vi "Value substituter in equations.vi"(1 "Cluster":T1={"All Param Names"=[], "All Param Values"=[], "Sp IDs"=[], "Sp States"=[], "Input Equations"=[], "CompID"=[], "CompSize"=[], "T-Sym"="time", "T"=0.0}) -> (0 "Output Equations":string[](array[string]))   [LabVIEW 2014]
doc: "This VI substitutes the numerical values of bio-model's parameters in its equations.\n\nDesigned by HB\nhaba@dtu.dk"
uses:
  ValSubsCtrl.ctl
panel:
  out "T 2":dbl
  out "CompSize 2":string[](array[string])
  out "T-Sym 2":string="time"
  out "CompID 2":string[](array[string])
  out "Input Equations 2":string[](array[string])
  out "All Param Names 2":string[](array[string])
  out "All Param Values 2":string[](array[string])
  out "Sp IDs 2":string[](array[string])
  out "Sp States 2":string[](array[string])
  out "operators (none)":string[](array[string])=["*", "+", "-", "/", "^", "(", ")"]
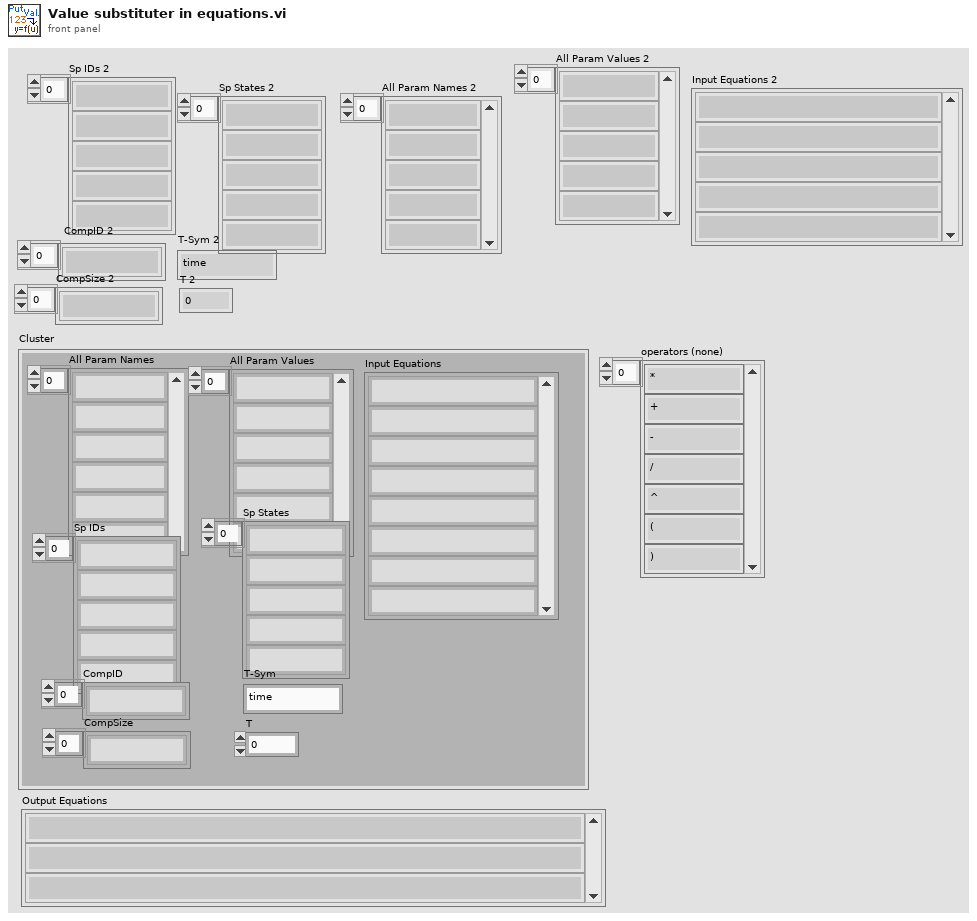
[diagram p1: front panel]
types:
  T1 = typedef "ValSubsCtrl.ctl" = cluster{"All Param Names":string[], "All Param Values":string[], "Sp IDs":string[], "Sp States":string[], "Input Equations":string[], "CompID":string[], "CompSize":string[], "T-Sym":string, "T":dbl}
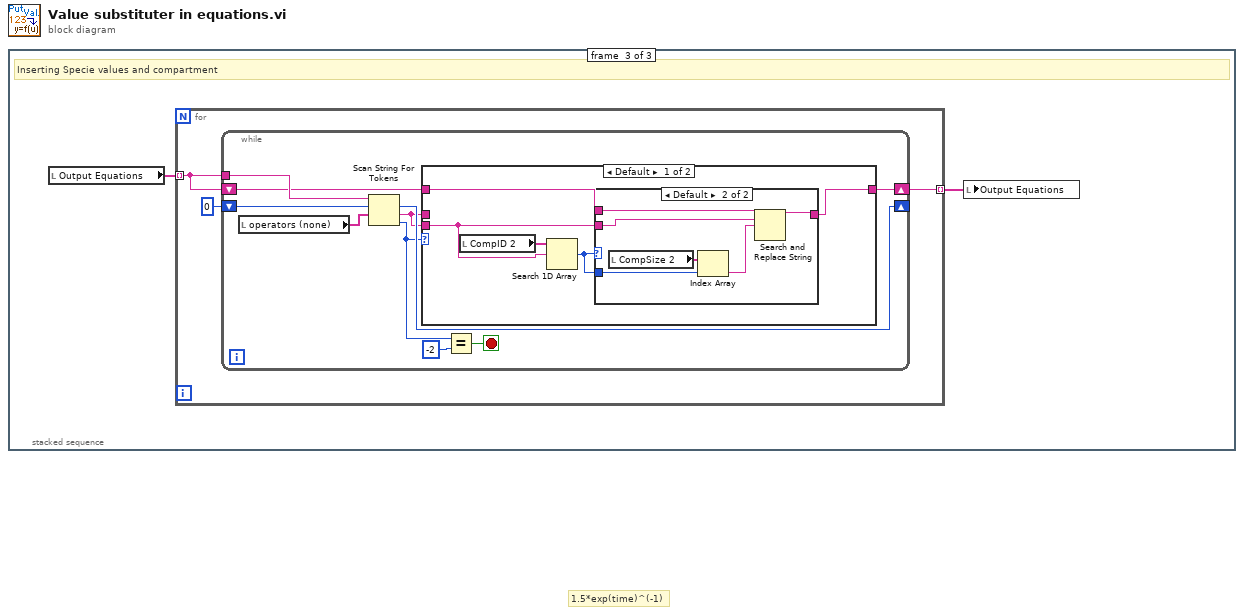
[diagram p0: block diagram]
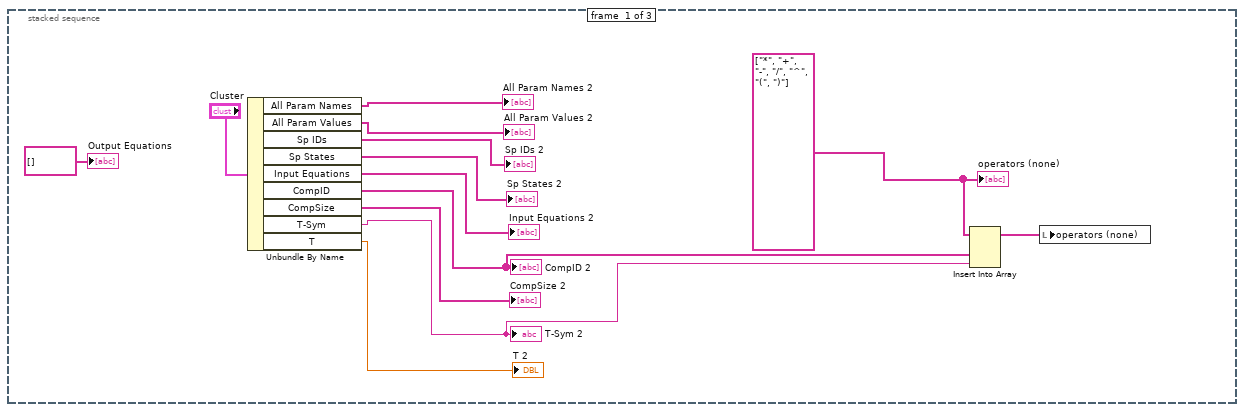
[diagram p2: hidden frame]
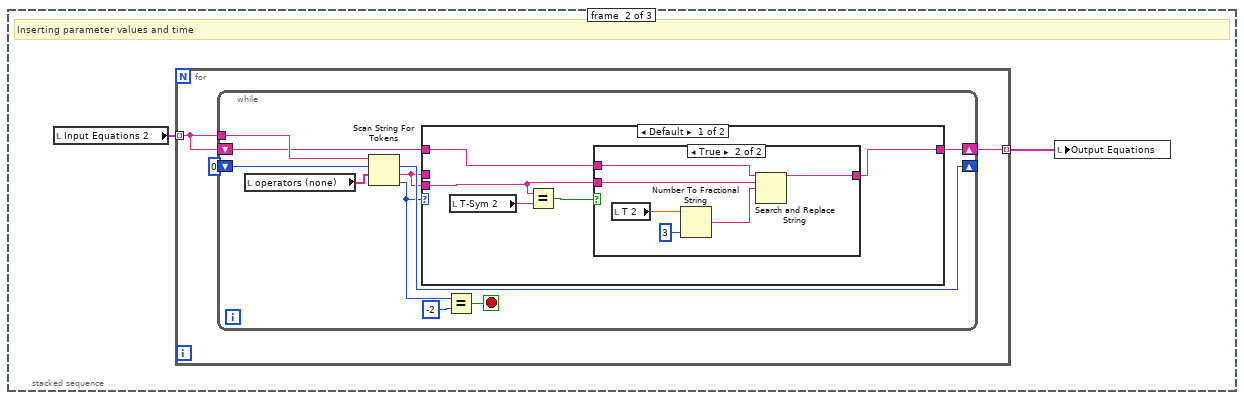
[diagram p3: hidden frame]
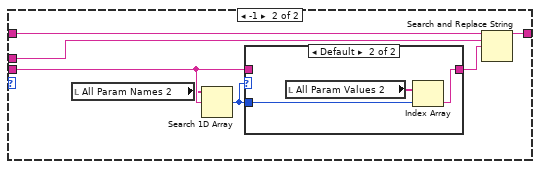
[diagram p5: hidden frame]
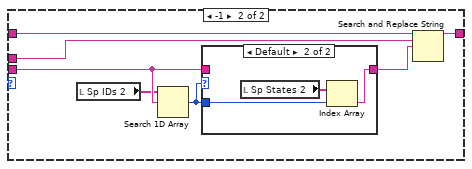
[diagram p8: hidden frame]
diagram:
  # "1.5*exp(time)^(-1)"
  n1 = stacked-sequence {
    frame #0 {
      w12 = string[] ["*", "+", "-", "/", "^", "(", ")"] ("operators (none)")
      n2 = Unbundle By Name("Cluster") -> ("All Param Names"=→"All Param Names 2":string[], "All Param Values"=→"All Param Values 2":string[], "Sp IDs"=→"Sp IDs 2":string[], "Sp States"=→"Sp States 2":string[], "Input Equations"=→"Input Equations 2":string[], "CompID"=w3:string[], "CompSize"=→"CompSize 2":string[], "T-Sym"=w2:string, "T"=→"T 2":dbl)
      "CompID 2" <- w3
      "T-Sym 2" <- w2
      n3 = Insert Into Array(array=w12, new element #1=w3, new element #2=w2) -> (w11:string[])  [unwired: 1 in]
      n4 = local write "operators (none)"(w11) -> ()
      "Output Equations" <- string[] [] ("Output Equations")
      "operators (none)" <- w12
    }
    frame #1 {
      # "Inserting parameter values and time"
      n5 = local read "Input Equations 2"() -> (w15:string[])
      n6 = for {
        tunnel: w15 -> [w17] mode=indexing
        tunnel: [w16] -> w14 mode=indexing
        n7 = while {
          shift-right: [w25] -> _
          shift-left: 0 ("offset past token") -> [w28]
          shift-right: [w20] -> w16
          shift-left: w17 -> [w21]
          tunnel: w17 -> [w22]
          stop <- w26 stop-if-true
          n8 = local read "operators (none)"() -> (w19:string[])
          n9 = Scan String For Tokens(7:w19, 8:w28, 9:w22) -> (0:w23:i32, 1:w24:string, 2:w25:i32)  [unwired: 3 in, 1 out]
          n10 = case shown="Default" w23 {
            tunnel: w24 -> [w29 w42]
            tunnel: w24 -> [_ w47]
            tunnel: [w32 w45] -> w20
            tunnel: w21 -> [w33 w44]
            frame Default {
              n11 = local read "T-Sym 2"() -> (w31:string)
              n12 = Equal?(x=w29, y=w31) -> (x = y?=w30:bool)
              n13 = case shown="True" w30 {
                tunnel: w33 -> [w34 w40]
                tunnel: [w34 w38] -> w32
                tunnel: w29 -> [_ w36]
                frame False {
                }
                frame True {
                  n14 = local read "T 2"() -> (w35:dbl)
                  n15 = Number To Fractional String(number=w35, precision (6)=i16 3) -> (F-format string=w39:string)  [unwired: 2 in]
                  n16 = Search and Replace String(input string=w40, search string=w36, replace string=w39) -> (result string=w38:string)  [unwired: 5 in, 3 out]
                }
              }
            }
            frame -1 {
              n17 = local read "All Param Names 2"() -> (w41:string[])
              n18 = Search 1D Array(1D array=w41, element=w42) -> (index of element=w43:i32)  [unwired: 1 in]
              n19 = case shown="Default" w43 {
                tunnel: [w48 w51] -> w46
                tunnel: w43 -> [_ w50]
                tunnel: w42 -> [w48 _]
                frame -1 {
                }
                frame Default {
                  n20 = local read "All Param Values 2"() -> (w49:string[])
                  n21 = Index Array(array=w49, index=w50) -> (element=w51:string)
                }
              }
              n22 = Search and Replace String(input string=w44, search string=w47, replace string=w46) -> (result string=w45:string)  [unwired: 5 in, 3 out]
            }
          }
          n23 = Equal?(x=w23, y=-2) -> (x = y?=w26:bool)
        }
      }
      n24 = local write "Output Equations"(w14) -> ()
    }
    frame #2 {
      # "Inserting Specie values and compartment"
      n25 = local read "Output Equations"() -> (w53:string[])
      n26 = for {
        tunnel: w53 -> [w55] mode=indexing
        tunnel: [w54] -> w52 mode=indexing
        n27 = while {
          shift-right: [w63] -> _
          shift-left: 0 ("offset past token") -> [w66]
          shift-right: [w58] -> w54
          shift-left: w55 -> [w59]
          tunnel: w55 -> [w60]
          stop <- w64 stop-if-true
          n28 = local read "operators (none)"() -> (w57:string[])
          n29 = Scan String For Tokens(7:w57, 8:w66, 9:w60) -> (0:w61:i32, 1:w62:string, 2:w63:i32)  [unwired: 3 in, 1 out]
          n30 = case shown="Default" w61 {
            tunnel: w62 -> [w67 w80]
            tunnel: w62 -> [_ w85]
            tunnel: [w68 w83] -> w58
            tunnel: w59 -> [w69 w82]
            frame Default {
              n31 = local read "CompID 2"() -> (w71:string[])
              n32 = Search 1D Array(1D array=w71, element=w67) -> (index of element=w70:i32)  [unwired: 1 in]
              n33 = case shown="Default" w70 {
                tunnel: [w72 w73] -> w68
                tunnel: w70 -> [_ w78]
                tunnel: w69 -> [w72 w76]
                tunnel: w67 -> [_ w75]
                frame -1 {
                }
                frame Default {
                  n34 = local read "CompSize 2"() -> (w77:string[])
                  n35 = Index Array(array=w77, index=w78) -> (element=w74:string)
                  n36 = Search and Replace String(input string=w76, search string=w75, replace string=w74) -> (result string=w73:string)  [unwired: 5 in, 3 out]
                }
              }
            }
            frame -1 {
              n37 = local read "Sp IDs 2"() -> (w79:string[])
              n38 = Search 1D Array(1D array=w79, element=w80) -> (index of element=w81:i32)  [unwired: 1 in]
              n39 = case shown="Default" w81 {
                tunnel: [w86 w89] -> w84
                tunnel: w81 -> [_ w88]
                tunnel: w80 -> [w86 _]
                frame -1 {
                }
                frame Default {
                  n40 = local read "Sp States 2"() -> (w87:string[])
                  n41 = Index Array(array=w87, index=w88) -> (element=w89:string)
                }
              }
              n42 = Search and Replace String(input string=w82, search string=w85, replace string=w84) -> (result string=w83:string)  [unwired: 5 in, 3 out]
            }
          }
          n43 = Equal?(x=w61, y=-2) -> (x = y?=w64:bool)
        }
      }
      n44 = local write "Output Equations"(w52) -> ()
    }
  }
